vi "Digitize.vi"(0 "Invert Polarity":bool, 1 "IF or Log":bool, 2 "# Sample/step":i32, 3 "ADC Rate (Hz)":i32, 4 "ADC Range":i32) -> (5 "mean":dbl, 6 "standard deviation":dbl)   [LabVIEW 2013]
uses:
  <vilib>/Analysis/NI_AALBase.lvlib
panel:
  out "ErrMsg":string
  # "Collects ADC data and calculates mean\nand standard deviation"
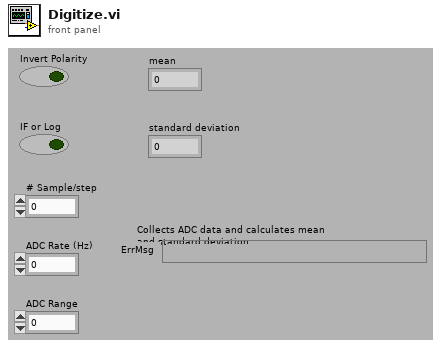
[diagram p1: front panel]
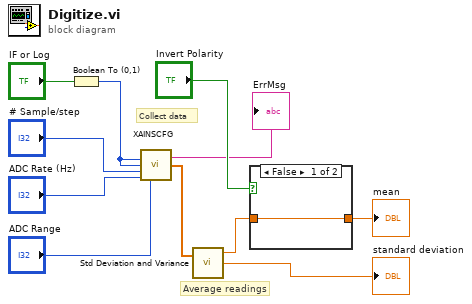
[diagram p0: block diagram]
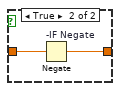
[diagram p2: hidden frame]
diagram:
  # "Collect data"
  # "Average readings"
  n1 = Boolean To (0,1)(Boolean="IF or Log") -> (0, 1=w4:i16)
  n2 = call "XAINSCFG.VI"("LowChan"=w4, "HighChan"=w4, "Count"="# Sample/step", "Rate"="ADC Rate (Hz)", "Range"="ADC Range") -> ("ErrMsg"=→"ErrMsg":string, "Voltage Data Array 2"=w5:sgl[])  [unwired: 7 in, 2 out]
  n3 = call <vilib>:"Std Deviation and Variance.vi"("X"=w5) -> ("mean"=w3:dbl, "standard deviation"=→"standard deviation":dbl)  [unwired: 1 in, 1 out]
  n4 = case shown="False" "Invert Polarity" {
    tunnel: [w12 w14] -> w2
    tunnel: w3 -> [w12 w13]
    frame False {
    }
    frame True {
      n5 = Negate "-IF Negate"(x=w13) -> (-x=w14:dbl)
    }
  }
  "mean" <- w2
